vi "QuantumX_DisableBlinking.vi"(8 "Error in":errorcluster, 10 "Signal":refnum<k24>, 11 "DevicesAndSignals":T1) -> (0 "Error out":errorcluster, 3 "DevicesAndSignals":T1)   [LabVIEW 2016]
doc: "Disables blinking at the connector to which the given signal belongs.\n\nSignal: Signal, whose connector should stop blinking."
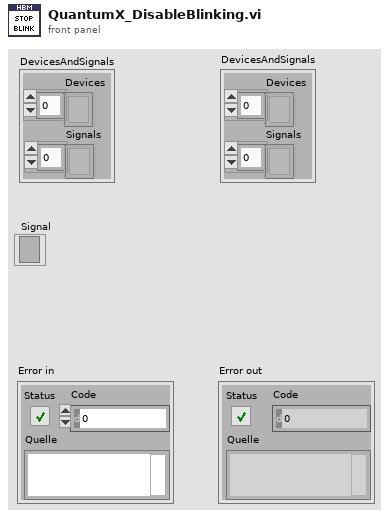
[diagram p1: front panel]
types:
  T1 = cluster{"Devices":refnum<k24>[], "Signals":refnum<k24>[]}
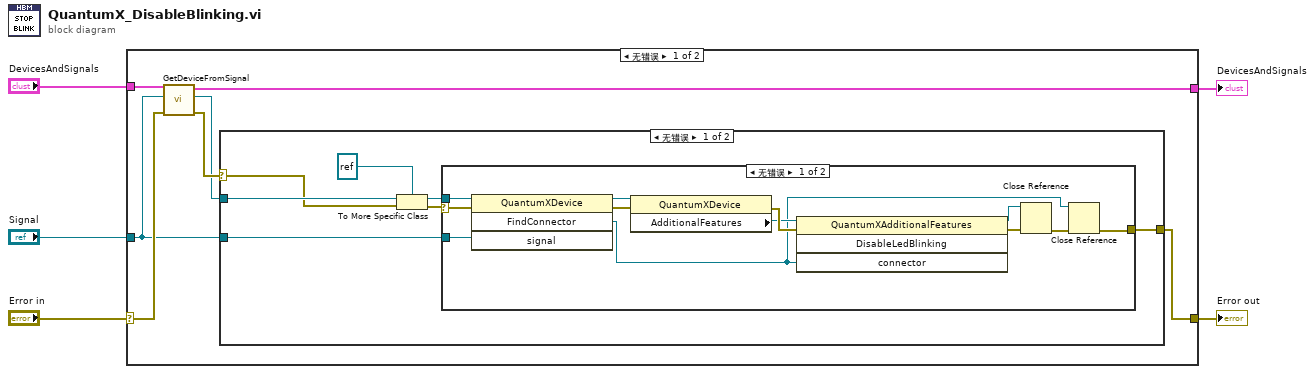
[diagram p0: block diagram]
diagram:
  n1 = case shown="无错误" "Error in" {
    selector: "Error in" -> [w11 w35]
    tunnel: "Signal" -> [w8 _]
    tunnel: "DevicesAndSignals" -> [w12 w34]
    tunnel: [w7 w35] -> w2
    tunnel: [w6 w34] -> w1
    frame No Error {
      n2 = call "GetDeviceFromSignal.vi"("Error in"=w11, "Signal"=w8, "DevicesAndSignals"=w12) -> ("Error out"=w10:errorcluster, "Device"=w9:refnum<k24>, "DevicesAndSignals"=w6:T1)  [unwired: 6 in]
      n3 = case shown="无错误" w10 {
        selector: w10 -> [w14 w33]
        tunnel: w9 -> [w18 _]
        tunnel: w8 -> [w16 _]
        tunnel: [w15 w33] -> w7
        frame No Error {
          n4 = To More Specific Class(target class=refnum<k24> refnum (".NET (Referenz)"), reference=w18, error in=w14) -> (specific class reference=w19:refnum<k24>, error out=w17:errorcluster)
          n5 = case shown="无错误" w17 {
            selector: w17 -> [w28 w32]
            tunnel: w19 -> [w29 _]
            tunnel: w16 -> [w27 _]
            tunnel: [w21 w32] -> w15
            frame No Error {
              n6 = invoke on="Methodenknoten" class="QuantumXDevice" method="FindConnector"(reference=w29, error in=w28, "signal"=w27) -> (reference out=w26:refnum<k24>, error out=w25:errorcluster, "FindConnector"=w20:refnum<k24>)  [unwired: 1 in, 1 out]
              n7 = property on="Eigenschaftsknoten" class="QuantumXDevice"(reference=w26, error in=w25) -> (error out=w31:errorcluster, "AdditionalFeatures"=w30:refnum<k24>)  [unwired: 1 out]
              n8 = invoke on="Methodenknoten" class="QuantumXAdditionalFeatures" method="DisableLedBlinking"(reference=w30, error in=w31, "connector"=w20) -> (reference out=w23:refnum<k24>, error out=w24:errorcluster)  [unwired: 1 in, 2 out]
              n9 = Close Reference(reference=w23, error in (no error)=w24) -> (error out=w22:errorcluster)
              n10 = Close Reference(reference=w20, error in (no error)=w22) -> (error out=w21:errorcluster)
            }
            frame Error {
            }
          }
        }
        frame Error {
        }
      }
    }
    frame Error {
    }
  }
  "Error out" <- w2
  "DevicesAndSignals" <- w1
